vi "Read Configuration.vi"(8 "error in (no error)":errorcluster, 11 "Micron Optics Driver in":refnum<class "Micron Optics Driver.lvclass">) -> (0 "error out":errorcluster, 2 "Configuration":T1={"Reference channel"=-1, "Detection Setting IDs"=[130, 130], "Address"="10.0.0.55", "Stream and average"=FALSE}, 3 "Micron Optics Driver out":refnum<class "Micron Optics Driver.lvclass">)   [LabVIEW 2016, in "Micron Optics Driver.lvclass"]
uses:
  Micron Optics Driver.lvclass
  C:/github/NHMFL_Core/Libraries/Instruments/Instrument Driver/Instrument Driver.lvclass
  Micron optics configuration.ctl
  Instrument Driver/Read User configuration.vi
panel:
  # "CH1\n.\n.\n.\n.\n.\nCH4"
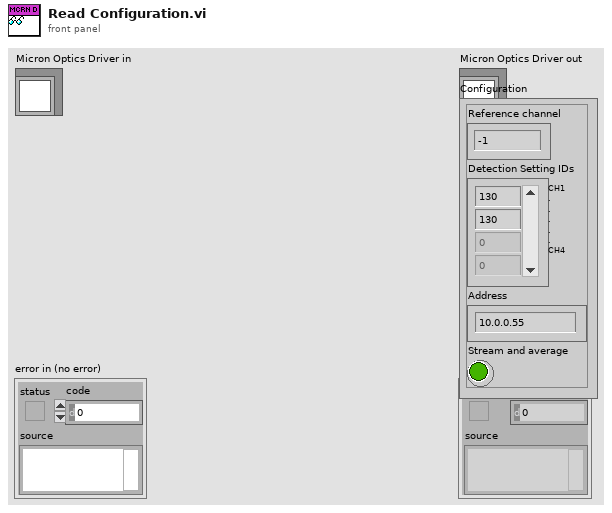
[diagram p1: front panel]
types:
  T1 = typedef "Micron optics configuration.ctl" = cluster{"Reference channel":i32, "Detection Setting IDs":u8[], "Address":string, "Stream and average":bool}
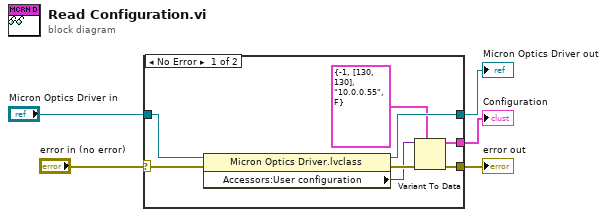
[diagram p0: block diagram]
diagram:
  n1 = case shown="No Error" "error in (no error)" {
    selector: "error in (no error)" -> [w13 w14]
    tunnel: [w9 w14] -> w4
    tunnel: [w11 w15] -> w2
    tunnel: "Micron Optics Driver in" -> [w12 w15]
    tunnel: [w6 _] -> w1
    frame No Error {
      n2 = property class="Micron Optics Driver.lvclass"(reference=w12, error in=w13) -> (reference out=w11:refnum<class "Micron Optics Driver.lvclass">, error out=w10:errorcluster, "Accessors:User configuration"=w8:variant)
      n3 = Variant To Data(error in=w10, type=T1 {"Reference channel"=-1, "Detection Setting IDs"=[130, 130], "Address"="10.0.0.55", "Stream and average"=FALSE} ("Configuration"), Variant=w8) -> (data=w6:T1, error out=w9:errorcluster)
    }
    frame Error {
    }
  }
  "error out" <- w4
  "Micron Optics Driver out" <- w2
  "Configuration" <- w1
